vi "74HC138.vi"(0 "A0":bool, 1 "A1":bool, 2 "A2":bool, 5 "S1":bool, 6 "S2`":bool, 7 "S3`":bool) -> (20 "Y0`":bool, 21 "Y1`":bool, 22 "Y2`":bool, 23 "Y3`":bool, 24 "Y4`":bool, 25 "Y5`":bool, 26 "Y6`":bool, 27 "Y7`":bool)   [LabVIEW 2018]
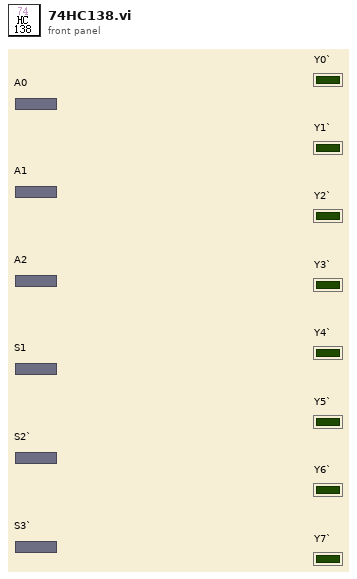
[diagram p1: front panel]
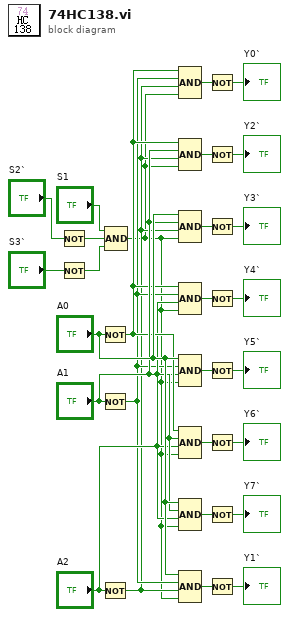
[diagram p0: block diagram]
diagram:
  n1 = Not(x="S2`") -> (.not. x?=w20:bool)
  n2 = Not(x="S3`") -> (.not. x?=w21:bool)
  n3 = Not(x="A0") -> (.not. x?=w26:bool)
  n4 = Not(x="A1") -> (.not. x?=w24:bool)
  n5 = Not(x="A2") -> (.not. x?=w23:bool)
  n6 = Compound Arithmetic op=AND ("复合运算")("S1", w20, w21) -> (w22:bool)
  n7 = Compound Arithmetic op=AND ("复合运算")(w26, w24, w23, w22) -> (w9:bool)
  n8 = Compound Arithmetic op=AND ("复合运算")(w26, "A1", w23, w22) -> (w11:bool)
  n9 = Compound Arithmetic op=AND ("复合运算")("A0", "A1", w23, w22) -> (w12:bool)
  n10 = Compound Arithmetic op=AND ("复合运算")(w26, w24, "A2", w22) -> (w13:bool)
  n11 = Compound Arithmetic op=AND ("复合运算")("A0", w24, "A2", w22) -> (w14:bool)
  n12 = Compound Arithmetic op=AND ("复合运算")(w26, "A1", "A2", w22) -> (w15:bool)
  n13 = Compound Arithmetic op=AND ("复合运算")("A0", "A1", "A2", w22) -> (w16:bool)
  n14 = Compound Arithmetic op=AND ("复合运算")("A0", w24, w23, w22) -> (w10:bool)
  n15 = Not(x=w9) -> (.not. x?=→"Y0`":bool)
  n16 = Not(x=w11) -> (.not. x?=→"Y2`":bool)
  n17 = Not(x=w12) -> (.not. x?=→"Y3`":bool)
  n18 = Not(x=w13) -> (.not. x?=→"Y4`":bool)
  n19 = Not(x=w14) -> (.not. x?=→"Y5`":bool)
  n20 = Not(x=w15) -> (.not. x?=→"Y6`":bool)
  n21 = Not(x=w16) -> (.not. x?=→"Y7`":bool)
  n22 = Not(x=w10) -> (.not. x?=→"Y1`":bool)
